vi "Set Refnum.vi"(8 "error in (no error)":errorcluster caption="entrée d'erreur (pas d'erreur)", 10 "Refnum":refnum<k24>, 11 "Cryptographic Hash_SHA256 en entrée":refnum<class "Cryptographic Hash_SHA256.lvclass">) -> (0 "error out":errorcluster caption="sortie d'erreur", 3 "Cryptographic Hash_SHA256 en sortie":refnum<class "Cryptographic Hash_SHA256.lvclass">)   [LabVIEW 2020, in "Library Cryptographic Hash.lvlib" / "Cryptographic Hash_SHA256.lvclass"]
uses:
  Cryptographic Hash_SHA256.lvclass
  Cryptographic Hash_SHA256.lvclass/Cryptographic Hash_SHA256.ctl
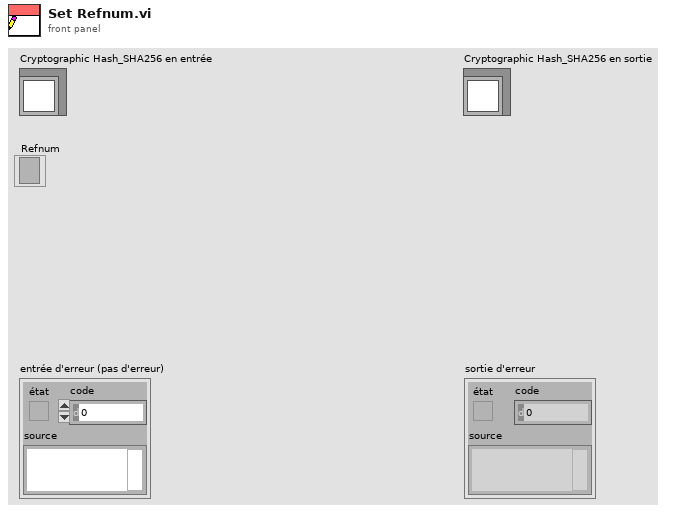
[diagram p1: front panel]
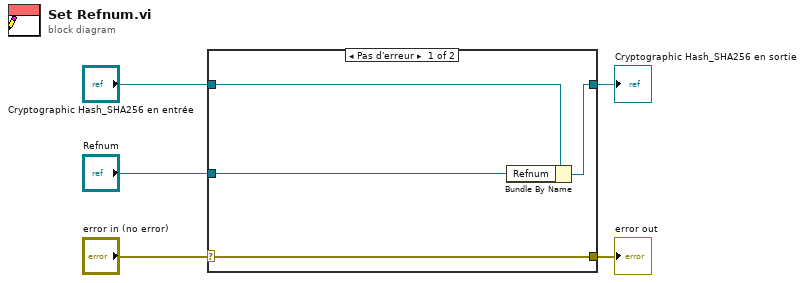
[diagram p0: block diagram]
diagram:
  n1 = case shown="Pas d'erreur" "error in (no error)" {
    selector: "error in (no error)" -> [w9 w10]
    tunnel: [w9 w10] -> w4
    tunnel: [w7 w11] -> w2
    tunnel: "Cryptographic Hash_SHA256 en entrée" -> [w8 w11]
    tunnel: "Refnum" -> [w6 _]
    frame No Error {
      n2 = Bundle By Name(cluster=w8, "Refnum"=w6) -> (w7:refnum<class "Cryptographic Hash_SHA256.lvclass">)
    }
    frame Error {
    }
  }
  "error out" <- w4
  "Cryptographic Hash_SHA256 en sortie" <- w2
